vi "Get part number info block from text file output line array.vi"(8 "error in (no error)":errorcluster, 10 "Key word":string, 11 "file (use dialog)":path) -> (0 "error out":errorcluster, 2 "Line array":string[](array[string]), 3 "Info block":string)   [LabVIEW 2013]
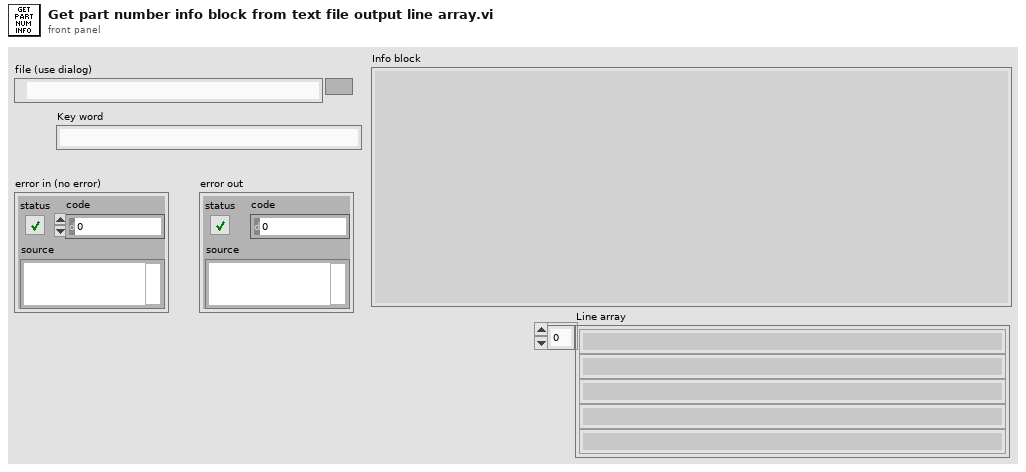
[diagram p1: front panel]
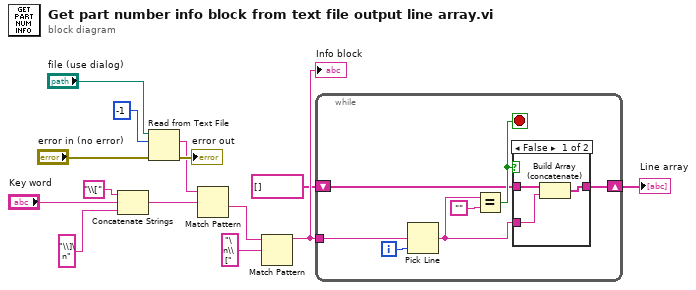
[diagram p0: block diagram]
diagram:
  n1 = Concatenate Strings("\\[" ("string"), "Key word", "\\]\n" ("string")) -> (w10:string)
  n2 = Read from Text File(file (use dialog)="file (use dialog)", count=-1, error in="error in (no error)") -> (text=w7:string, error out=→"error out":errorcluster)  [unwired: 1 in, 2 out]
  n3 = Match Pattern(string=w7, regular expression=w10) -> (after substring=w11:string)  [unwired: 1 in, 3 out]
  n4 = Match Pattern(string=w11, regular expression="\n\\[") -> (before substring=w3:string)  [unwired: 1 in, 3 out]
  "Info block" <- w3
  n5 = while {
    tunnel: w3 -> [w20]
    shift-right: [w15] -> w1
    shift-left: string[] [] -> [w17]
    i -> [w21]
    stop <- w18 stop-if-true
    n6 = Pick Line(multi-line string=w20, line index=w21) -> (output string=w16:string)  [unwired: 1 in]
    n7 = Equal?(x=w16, y="") -> (x = y?=w18:bool)
    n8 = case shown="False" w18 {
      tunnel: w17 -> [w24 w25]
      tunnel: w16 -> [w23 _]
      tunnel: [w22 w25] -> w15
      frame False {
        n9 = Build Array (concatenate)(w24, w23) -> (w22:string[])
      }
      frame True {
      }
    }
  }
  "Line array" <- w1
